vi "CalculateDelay_2chan.vi"(8 "input valid":bool=TRUE, 9 "cos_fi":fxp<+/-,16,0>, 10 "sin fi":fxp<+/-,16,0>, 11 "Data in":fxp<+/-,16,14>[](array[numeric])=[0.0, 0.0, 0.0, 0.0]) -> (0 "output valid":bool, 3 "Data out":fxp<+/-,16,14>[](array[numeric]))   [LabVIEW 2013]
doc: "Calculates various combinations on I_in, Q_in and cos(fi) and sin(fi) to be used later to delay the output signal"
uses:
  <vilib>/rvi/FXPMathLib/FxpInterpret/XNode/nifxpmath_Interpret.xnode
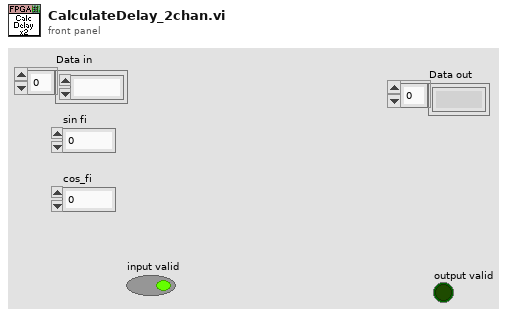
[diagram p1: front panel]
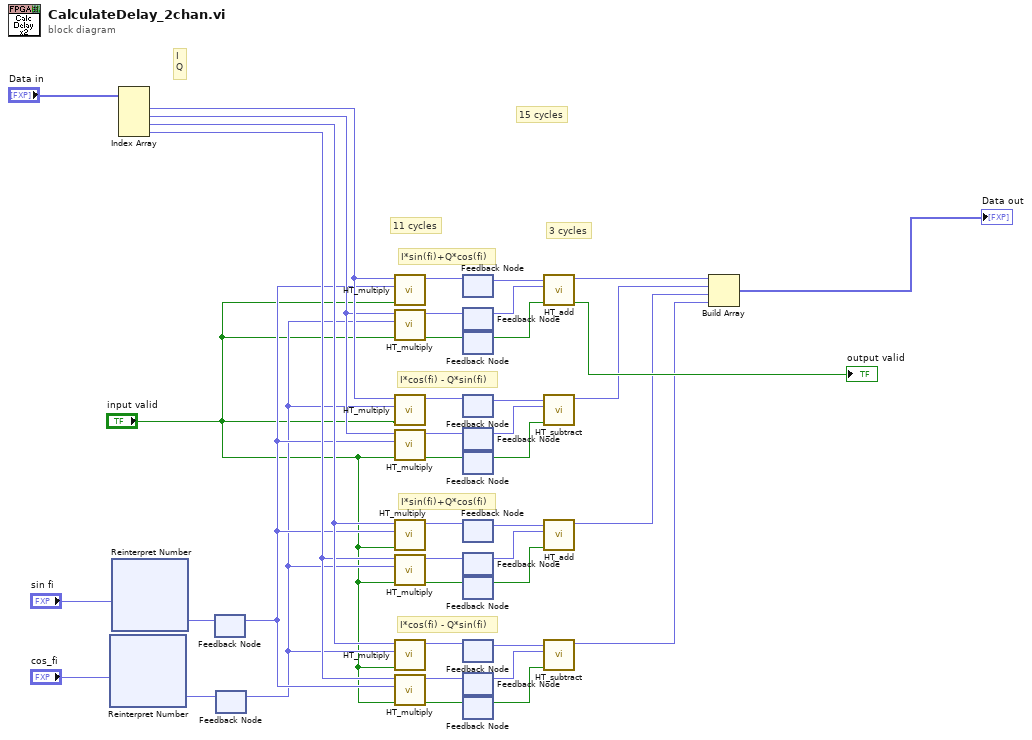
[diagram p0: block diagram]
diagram:
  # "3 cycles"
  # "11 cycles"
  # "15 cycles"
  # "I*cos(fi) - Q*sin(fi)"
  # "I*sin(fi)+Q*cos(fi)"
  # "I*cos(fi) - Q*sin(fi)"
  # "I\nQ"
  # "I*sin(fi)+Q*cos(fi)"
  n1 = xnode "Reinterpret Number"("x"="cos_fi") -> ("y"=w22:fxp<+/-,16,2>)
  n2 = xnode "Reinterpret Number"("x"="sin fi") -> ("y"=w23:fxp<+/-,16,2>)
  n3 = Index Array(array="Data in") -> (element #1=w29:fxp<+/-,16,14>, element #2=w28:fxp<+/-,16,14>, element #3=w7:fxp<+/-,16,14>, element #4=w6:fxp<+/-,16,14>)  [unwired: 4 in]
  n4 = feedback #1() -> (w5:fxp<+/-,16,2>)  [unwired: 1 in]
  n5 = feedback-in #1(w23) -> ()
  n6 = feedback #2() -> (w4:fxp<+/-,16,2>)  [unwired: 1 in]
  n7 = feedback-in #2(w22) -> ()
  n8 = call "HT_multiply.vi"("input valid"="input valid", "y"=w5, "x"=w29) -> ("x*y"=w41:fxp<+/-,16,14>)  [unwired: 7 in, 1 out]
  n9 = call "HT_multiply.vi"("input valid"="input valid", "y"=w4, "x"=w28) -> ("output valid"=w36:bool, "x*y"=w38:fxp<+/-,16,14>)  [unwired: 7 in]
  n10 = call "HT_multiply.vi"("input valid"="input valid", "y"=w4, "x"=w29) -> ("x*y"=w30:fxp<+/-,16,14>)  [unwired: 7 in, 1 out]
  n11 = call "HT_multiply.vi"("input valid"="input valid", "y"=w5, "x"=w28) -> ("output valid"=w35:bool, "x*y"=w33:fxp<+/-,16,14>)  [unwired: 7 in]
  n12 = call "HT_multiply.vi"("input valid"="input valid", "y"=w5, "x"=w7) -> ("x*y"=w8:fxp<+/-,16,14>)  [unwired: 7 in, 1 out]
  n13 = call "HT_multiply.vi"("input valid"="input valid", "y"=w4, "x"=w6) -> ("output valid"=w13:bool, "x*y"=w11:fxp<+/-,16,14>)  [unwired: 7 in]
  n14 = call "HT_multiply.vi"("input valid"="input valid", "y"=w4, "x"=w7) -> ("x*y"=w19:fxp<+/-,16,14>)  [unwired: 7 in, 1 out]
  n15 = call "HT_multiply.vi"("input valid"="input valid", "y"=w5, "x"=w6) -> ("output valid"=w14:bool, "x*y"=w16:fxp<+/-,16,14>)  [unwired: 7 in]
  n16 = feedback #3() -> (w40:fxp<+/-,16,14>)  [unwired: 1 in]
  n17 = feedback-in #3(w41) -> ()
  n18 = feedback #4() -> (w37:fxp<+/-,16,14>)  [unwired: 1 in]
  n19 = feedback-in #4(w38) -> ()
  n20 = feedback #5() -> (w39:bool)  [unwired: 1 in]
  n21 = feedback-in #5(w36) -> ()
  n22 = feedback #6() -> (w31:fxp<+/-,16,14>)  [unwired: 1 in]
  n23 = feedback-in #6(w30) -> ()
  n24 = feedback #7() -> (w34:fxp<+/-,16,14>)  [unwired: 1 in]
  n25 = feedback-in #7(w33) -> ()
  n26 = feedback #8() -> (w32:bool)  [unwired: 1 in]
  n27 = feedback-in #8(w35) -> ()
  n28 = feedback #9() -> (w9:fxp<+/-,16,14>)  [unwired: 1 in]
  n29 = feedback-in #9(w8) -> ()
  n30 = feedback #10() -> (w12:fxp<+/-,16,14>)  [unwired: 1 in]
  n31 = feedback-in #10(w11) -> ()
  n32 = feedback #11() -> (w10:bool)  [unwired: 1 in]
  n33 = feedback-in #11(w13) -> ()
  n34 = feedback #12() -> (w18:fxp<+/-,16,14>)  [unwired: 1 in]
  n35 = feedback-in #12(w19) -> ()
  n36 = feedback #13() -> (w15:fxp<+/-,16,14>)  [unwired: 1 in]
  n37 = feedback-in #13(w16) -> ()
  n38 = feedback #14() -> (w17:bool)  [unwired: 1 in]
  n39 = feedback-in #14(w14) -> ()
  n40 = call "HT_add.vi"("input valid"=w39, "y"=w37, "x"=w40) -> ("output valid"=→"output valid":bool, "x+y"=w20:fxp<+/-,16,14>)  [unwired: 7 in]
  n41 = call "HT_subtract.vi"("input valid"=w32, "y"=w34, "x"=w31) -> ("x+y"=w21:fxp<+/-,16,14>)  [unwired: 7 in, 1 out]
  n42 = call "HT_add.vi"("input valid"=w10, "y"=w12, "x"=w9) -> ("x+y"=w3:fxp<+/-,16,14>)  [unwired: 7 in, 1 out]
  n43 = call "HT_subtract.vi"("input valid"=w17, "y"=w15, "x"=w18) -> ("x+y"=w2:fxp<+/-,16,14>)  [unwired: 7 in, 1 out]
  n44 = Build Array(w20, w21, w3, w2) -> (→"Data out":fxp<+/-,16,14>[])
